vi "inputOLD.vi"(8 "error in":errorcluster, 9 "result allocation":T1, 10 "parameters":T1, 11 "module in":refnum<class "current tag file io module runtime.lvclass">) -> (0 "error out":errorcluster, 1 "results":T1, 2 "parameter allocation":T1, 3 "module out":refnum<class "current tag file io module runtime.lvclass">)   [LabVIEW 2013, in "current tag file io module runtime.lvclass"]
doc: "Provides an interface for information processing by a module at runtime. While this interface performs no operations, a child should provide an override which may process data in any manner necessary."
uses:
  current tag file io module runtime.lvclass
  <vilib>/NI/Tag Bus/table/data table.lvlib
  <vilib>/NI/Tag Bus/table/data polymorphs/read one/read Double.vi
  <vilib>/NI/Tag Bus/table/data polymorphs/write one/write Double.vi
  <vilib>/NI/Tag Bus/table/data polymorphs/read one/read Boolean.vi
  <vilib>/NI/Tag Bus/table/data polymorphs/write one/write Array of String.vi
  <vilib>/NI/Tag Bus/table/data polymorphs/read one/read Array of String.vi
  <vilib>/NI/Tag Bus/table/data polymorphs/read one/read Single.vi
  <vilib>/NI/Tag Bus/table/data polymorphs/write one/write Single.vi
  <vilib>/NI/Tag Bus/table/data polymorphs/read one/read I64.vi
  <vilib>/NI/Tag Bus/table/data polymorphs/write one/write I64.vi
  <vilib>/NI/Tag Bus/table/data polymorphs/read one/read I32.vi
  <vilib>/NI/Tag Bus/table/data polymorphs/write one/write I32.vi
  <vilib>/NI/Tag Bus/table/data polymorphs/read one/read I16.vi
  <vilib>/NI/Tag Bus/table/data polymorphs/write one/write I16.vi
  <vilib>/NI/Tag Bus/table/data polymorphs/read one/read I8.vi
  <vilib>/NI/Tag Bus/table/data polymorphs/write one/write I8.vi
  <vilib>/NI/Tag Bus/table/data polymorphs/read one/read U64.vi
  <vilib>/NI/Tag Bus/table/data polymorphs/write one/write U64.vi
  <vilib>/NI/Tag Bus/table/data polymorphs/read one/read U32.vi
  <vilib>/NI/Tag Bus/table/data polymorphs/write one/write U32.vi
  <vilib>/NI/Tag Bus/table/data polymorphs/read one/read U16.vi
  <vilib>/NI/Tag Bus/table/data polymorphs/write one/write U16.vi
  <vilib>/NI/Tag Bus/table/data polymorphs/read one/read U8.vi
  <vilib>/NI/Tag Bus/table/data polymorphs/write one/write U8.vi
  <vilib>/NI/Tag Bus/table/data polymorphs/write one/write Boolean.vi
  <vilib>/NI/Tag Bus/table/data polymorphs/read one/read String.vi
  <vilib>/NI/Tag Bus/table/data polymorphs/write one/write String.vi
  <vilib>/NI/Tag Bus/table/data polymorphs/read one/read Array of Double.vi
  <vilib>/NI/Tag Bus/table/data polymorphs/write one/write Array of Double.vi
  <vilib>/NI/Tag Bus/table/data polymorphs/read one/read Array of Single.vi
  <vilib>/NI/Tag Bus/table/data polymorphs/write one/write Array of Single.vi
  <vilib>/NI/Tag Bus/table/data polymorphs/read one/read Array of I64.vi
  <vilib>/NI/Tag Bus/table/data polymorphs/write one/write Array of I64.vi
  <vilib>/NI/Tag Bus/table/data polymorphs/read one/read Array of I32.vi
  <vilib>/NI/Tag Bus/table/data polymorphs/write one/write Array of I32.vi
  <vilib>/NI/Tag Bus/table/data polymorphs/read one/read Array of I16.vi
  <vilib>/NI/Tag Bus/table/data polymorphs/write one/write Array of I16.vi
  <vilib>/NI/Tag Bus/table/data polymorphs/read one/read Array of I8.vi
  <vilib>/NI/Tag Bus/table/data polymorphs/write one/write Array of I8.vi
  <vilib>/NI/Tag Bus/table/data polymorphs/read one/read Array of U64.vi
  <vilib>/NI/Tag Bus/table/data polymorphs/write one/write Array of U64.vi
  <vilib>/NI/Tag Bus/table/data polymorphs/read one/read Array of U32.vi
  <vilib>/NI/Tag Bus/table/data polymorphs/write one/write Array of U32.vi
  <vilib>/NI/Tag Bus/table/data polymorphs/read one/read Array of U16.vi
  <vilib>/NI/Tag Bus/table/data polymorphs/write one/write Array of U16.vi
  <vilib>/NI/Tag Bus/table/data polymorphs/read one/read Array of U8.vi
  <vilib>/NI/Tag Bus/table/data polymorphs/write one/write Array of U8.vi
  <vilib>/NI/Tag Bus/table/data polymorphs/read one/read Array of Boolean.vi
  <vilib>/NI/Tag Bus/table/data polymorphs/write one/write Array of Boolean.vi
  <vilib>/NI/Tag Bus/table/data table.ctl
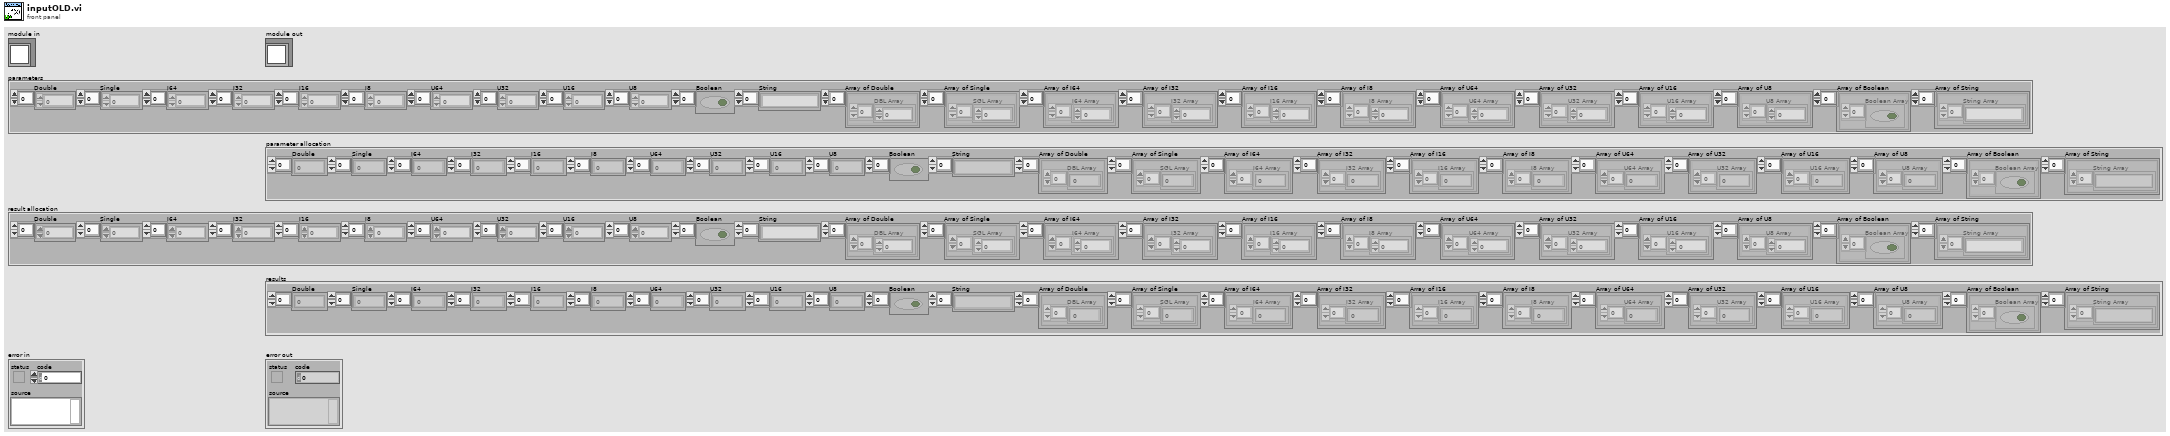
[diagram p1: front panel]
types:
  T1 = typedef "tag bus.lvlib/data table.lvlib/data table.ctl" = cluster{"Double":dbl[], "Single":sgl[], "I64":i64[], "I32":i32[], "I16":i16[], "I8":i8[], "U64":u64[], "U32":u32[], "U16":u16[], "U8":u8[], "Boolean":bool[], "String":string[], "Array of Double":cluster{"DBL Array":dbl[]}[], "Array of Single":cluster{"SGL Array":sgl[]}[], "Array of I64":cluster{"I64 Array":i64[]}[], "Array of I32":cluster{"I32 Array":i32[]}[], "Array of I16":cluster{"I16 Array":i16[]}[], "Array of I8":cluster{"I8 Array":i8[]}[], "Array of U64":cluster{"U64 Array":u64[]}[], "Array of U32":cluster{"U32 Array":u32[]}[], "Array of U16":cluster{"U16 Array":u16[]}[], "Array of U8":cluster{"U8 Array":u8[]}[], "Array of Boolean":cluster{"Boolean Array":bool[]}[], "Array of String":cluster{"String Array":string[]}[]}
  T2 = typedef "current tag file io module runtime.lvclass/current tag file io configuration.ctl" = cluster{"index":i32, "data type":T3, "refnum":refnum<file>}
  T3 = typedef "tag bus.lvlib/tag descriptor.lvclass/Data Type.ctl" = enum16{"Double", "Single", "I64", "I32", "I16", "I8", "U64", "U32", "U16", "U8", "Boolean", "String", "Array of Double", "Array of Single", "Array of I64", "Array of I32", "Array of I16", "Array of I8", "Array of U64", "Array of U32", "Array of U16", "Array of U8", "Array of Boolean", "Array of String"}
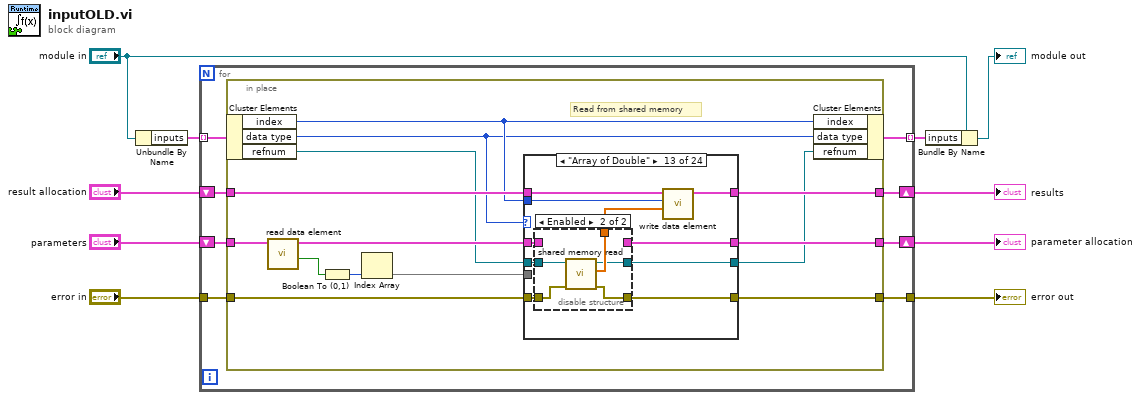
[diagram p0: block diagram]
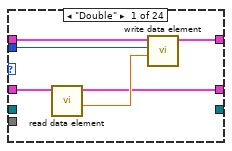
[diagram p2: hidden frame]
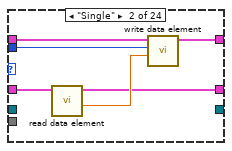
[diagram p3: hidden frame]
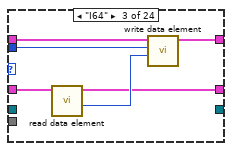
[diagram p4: hidden frame]
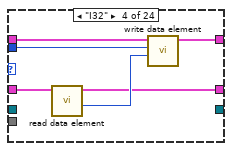
[diagram p5: hidden frame]
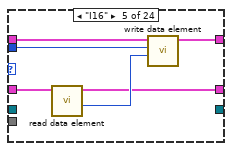
[diagram p6: hidden frame]
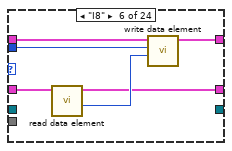
[diagram p7: hidden frame]
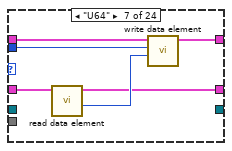
[diagram p8: hidden frame]
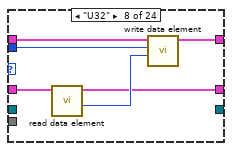
[diagram p9: hidden frame]
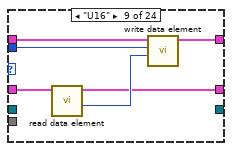
[diagram p10: hidden frame]
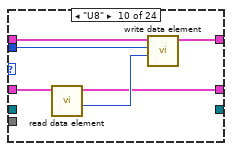
[diagram p11: hidden frame]
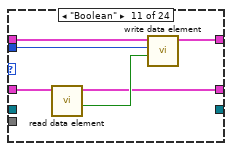
[diagram p12: hidden frame]
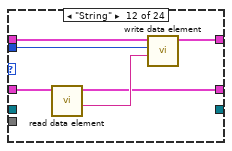
[diagram p13: hidden frame]
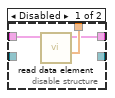
[diagram p14: hidden frame]
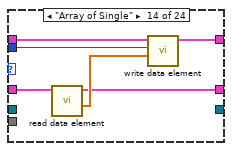
[diagram p15: hidden frame]
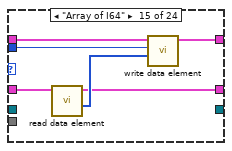
[diagram p16: hidden frame]
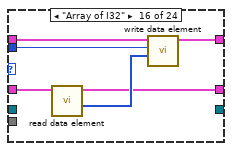
[diagram p17: hidden frame]
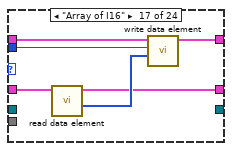
[diagram p18: hidden frame]
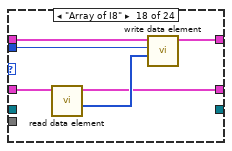
[diagram p19: hidden frame]
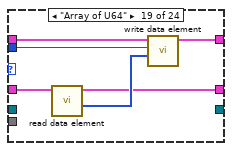
[diagram p20: hidden frame]
diagram:
  n1 = Unbundle By Name("module in") -> ("inputs"=w8:T2[])
  n2 = for {
    tunnel: w8 -> [w18] mode=indexing
    tunnel: [w17] -> w7 mode=indexing
    shift-right: [w13] -> w5
    shift-left: "parameters" -> [w16]
    shift-right: [w14] -> w3
    shift-left: "result allocation" -> [w15]
    tunnel: "error in" -> [w12]
    tunnel: [w11] -> w1
    n3 = in-place {
      in-place-border: w16 -> [w32]
      in-place-border: w15 -> [w31]
      in-place-border: [w30] -> w14
      in-place-border: [w25] -> w13
      in-place-border: w12 -> [w21]
      in-place-border: [w19] -> w11
      # "Read from shared memory"
      n4 = in-place-cluster #1(w18) -> ("index"=w24:i32, "data type"=w23:T3, "refnum"=w22:refnum<file>)
      n5 = call-poly <vilib>:"read data element.vi"("data table in"=w32) -> ("value"=w28:bool, "data table out"=w26:T1)  [unwired: 9 in]
      n6 = Boolean To (0,1)(Boolean=w28) -> (0, 1=w29:i16)
      n7 = Index Array(index=w29) -> (element=w27)  [unwired: 1 in]
      n8 = case shown="\"Array of Double\"" w23 {
        tunnel: w31 -> [w33 w39 w45 w51 w57 w63 w69 w75 w81 w87 w93 w99 w109 w123 w129 w135 w141 w147 w153 w159 w165 w171 w177 w183]
        tunnel: [w38 w44 w50 w56 w62 w68 w74 w80 w86 w92 w98 w104 w114 w128 w134 w140 w146 w152 w158 w164 w170 w176 w182 w188] -> w30
        tunnel: w27 -> [_ _ _ _ _ _ _ _ _ _ _ _ _ _ _ _ _ _ _ _ _ _ _ _]
        tunnel: w24 -> [w37 w43 w49 w55 w61 w67 w73 w79 w85 w91 w97 w103 w113 w127 w133 w139 w145 w151 w157 w163 w169 w175 w181 w187]
        tunnel: w26 -> [w35 w41 w47 w53 w59 w65 w71 w77 w83 w89 w95 w101 w111 w125 w131 w137 w143 w149 w155 w161 w167 w173 w179 w185]
        tunnel: [w34 w40 w46 w52 w58 w64 w70 w76 w82 w88 w94 w100 w110 w124 w130 w136 w142 w148 w154 w160 w166 w172 w178 w184] -> w25
        tunnel: w22 -> [_ _ _ _ _ _ _ _ _ _ _ _ w108 _ _ _ _ _ _ _ _ _ _ _]
        tunnel: w21 -> [_ _ _ _ _ _ _ _ _ _ _ _ w107 _ _ _ _ _ _ _ _ _ _ _]
        tunnel: [_ _ _ _ _ _ _ _ _ _ _ _ w106 _ _ _ _ _ _ _ _ _ _ _] -> w20
        tunnel: [_ _ _ _ _ _ _ _ _ _ _ _ w105 _ _ _ _ _ _ _ _ _ _ _] -> w19
        frame "Double" {
          n9 = call-poly <vilib>:"read data element.vi"("data table in"=w35) -> ("value"=w36:dbl, "data table out"=w34:T1)  [unwired: 9 in]
          n10 = call-poly <vilib>:"write data element.vi"("value"=w36, "index"=w37, "data table in"=w33) -> ("data table out"=w38:T1)  [unwired: 8 in]
        }
        frame "Single" {
          n11 = call-poly <vilib>:"read data element.vi"("data table in"=w41) -> ("value"=w42:sgl, "data table out"=w40:T1)  [unwired: 9 in]
          n12 = call-poly <vilib>:"write data element.vi"("value"=w42, "index"=w43, "data table in"=w39) -> ("data table out"=w44:T1)  [unwired: 8 in]
        }
        frame "I64" {
          n13 = call-poly <vilib>:"read data element.vi"("data table in"=w47) -> ("value"=w48:i64, "data table out"=w46:T1)  [unwired: 9 in]
          n14 = call-poly <vilib>:"write data element.vi"("value"=w48, "index"=w49, "data table in"=w45) -> ("data table out"=w50:T1)  [unwired: 8 in]
        }
        frame "I32" {
          n15 = call-poly <vilib>:"read data element.vi"("data table in"=w53) -> ("value"=w54:i32, "data table out"=w52:T1)  [unwired: 9 in]
          n16 = call-poly <vilib>:"write data element.vi"("value"=w54, "index"=w55, "data table in"=w51) -> ("data table out"=w56:T1)  [unwired: 8 in]
        }
        frame "I16" {
          n17 = call-poly <vilib>:"read data element.vi"("data table in"=w59) -> ("value"=w60:i16, "data table out"=w58:T1)  [unwired: 9 in]
          n18 = call-poly <vilib>:"write data element.vi"("value"=w60, "index"=w61, "data table in"=w57) -> ("data table out"=w62:T1)  [unwired: 8 in]
        }
        frame "I8" {
          n19 = call-poly <vilib>:"read data element.vi"("data table in"=w65) -> ("value"=w66:i8, "data table out"=w64:T1)  [unwired: 9 in]
          n20 = call-poly <vilib>:"write data element.vi"("value"=w66, "index"=w67, "data table in"=w63) -> ("data table out"=w68:T1)  [unwired: 8 in]
        }
        frame "U64" {
          n21 = call-poly <vilib>:"read data element.vi"("data table in"=w71) -> ("value"=w72:u64, "data table out"=w70:T1)  [unwired: 9 in]
          n22 = call-poly <vilib>:"write data element.vi"("value"=w72, "index"=w73, "data table in"=w69) -> ("data table out"=w74:T1)  [unwired: 8 in]
        }
        frame "U32" {
          n23 = call-poly <vilib>:"read data element.vi"("data table in"=w77) -> ("value"=w78:u32, "data table out"=w76:T1)  [unwired: 9 in]
          n24 = call-poly <vilib>:"write data element.vi"("value"=w78, "index"=w79, "data table in"=w75) -> ("data table out"=w80:T1)  [unwired: 8 in]
        }
        frame "U16" {
          n25 = call-poly <vilib>:"read data element.vi"("data table in"=w83) -> ("value"=w84:u16, "data table out"=w82:T1)  [unwired: 9 in]
          n26 = call-poly <vilib>:"write data element.vi"("value"=w84, "index"=w85, "data table in"=w81) -> ("data table out"=w86:T1)  [unwired: 8 in]
        }
        frame "U8" {
          n27 = call-poly <vilib>:"read data element.vi"("data table in"=w89) -> ("value"=w90:u8, "data table out"=w88:T1)  [unwired: 9 in]
          n28 = call-poly <vilib>:"write data element.vi"("value"=w90, "index"=w91, "data table in"=w87) -> ("data table out"=w92:T1)  [unwired: 8 in]
        }
        frame "Boolean" {
          n29 = call-poly <vilib>:"read data element.vi"("data table in"=w95) -> ("value"=w96:bool, "data table out"=w94:T1)  [unwired: 9 in]
          n30 = call-poly <vilib>:"write data element.vi"("value"=w96, "index"=w97, "data table in"=w93) -> ("data table out"=w98:T1)  [unwired: 8 in]
        }
        frame "String" {
          n31 = call-poly <vilib>:"read data element.vi"("data table in"=w101) -> ("value"=w102:string, "data table out"=w100:T1)  [unwired: 9 in]
          n32 = call-poly <vilib>:"write data element.vi"("value"=w102, "index"=w103, "data table in"=w99) -> ("data table out"=w104:T1)  [unwired: 8 in]
        }
        frame "Array of Double" {
          n33 = disable-structure shown="Enabled" {
            disable-tunnel: [w117 w122] -> w112
            disable-tunnel: w111 -> [w116 _]
            disable-tunnel: [w115 _] -> w110
            disable-tunnel: w108 -> [_ w121]
            disable-tunnel: w107 -> [_ w120]
            disable-tunnel: [_ w119] -> w106
            disable-tunnel: [_ w118] -> w105
            frame Disabled {
              n34 = call-poly <vilib>:"read data element.vi"("data table in"=w116) -> ("value"=w117:dbl[], "data table out"=w115:T1)  [unwired: 9 in]
            }
            frame Enabled {
              n35 = call "shared memory read.vi"("error in"=w120, "refnum in"=w121) -> ("error out"=w118:errorcluster, "Data Array out"=w122:dbl[], "refnum out"=w119:refnum<file>)  [unwired: 6 in, 1 out]
            }
          }
          n36 = call-poly <vilib>:"write data element.vi"("value"=w112, "index"=w113, "data table in"=w109) -> ("data table out"=w114:T1)  [unwired: 8 in]
        }
        frame "Array of Single" {
          n37 = call-poly <vilib>:"read data element.vi"("data table in"=w125) -> ("value"=w126:sgl[], "data table out"=w124:T1)  [unwired: 9 in]
          n38 = call-poly <vilib>:"write data element.vi"("value"=w126, "index"=w127, "data table in"=w123) -> ("data table out"=w128:T1)  [unwired: 8 in]
        }
        frame "Array of I64" {
          n39 = call-poly <vilib>:"read data element.vi"("data table in"=w131) -> ("value"=w132:i64[], "data table out"=w130:T1)  [unwired: 9 in]
          n40 = call-poly <vilib>:"write data element.vi"("value"=w132, "index"=w133, "data table in"=w129) -> ("data table out"=w134:T1)  [unwired: 8 in]
        }
        frame "Array of I32" {
          n41 = call-poly <vilib>:"read data element.vi"("data table in"=w137) -> ("value"=w138:i32[], "data table out"=w136:T1)  [unwired: 9 in]
          n42 = call-poly <vilib>:"write data element.vi"("value"=w138, "index"=w139, "data table in"=w135) -> ("data table out"=w140:T1)  [unwired: 8 in]
        }
        frame "Array of I16" {
          n43 = call-poly <vilib>:"read data element.vi"("data table in"=w143) -> ("value"=w144:i16[], "data table out"=w142:T1)  [unwired: 9 in]
          n44 = call-poly <vilib>:"write data element.vi"("value"=w144, "index"=w145, "data table in"=w141) -> ("data table out"=w146:T1)  [unwired: 8 in]
        }
        frame "Array of I8" {
          n45 = call-poly <vilib>:"read data element.vi"("data table in"=w149) -> ("value"=w150:i8[], "data table out"=w148:T1)  [unwired: 9 in]
          n46 = call-poly <vilib>:"write data element.vi"("value"=w150, "index"=w151, "data table in"=w147) -> ("data table out"=w152:T1)  [unwired: 8 in]
        }
        frame "Array of U64" {
          n47 = call-poly <vilib>:"read data element.vi"("data table in"=w155) -> ("value"=w156:u64[], "data table out"=w154:T1)  [unwired: 9 in]
          n48 = call-poly <vilib>:"write data element.vi"("value"=w156, "index"=w157, "data table in"=w153) -> ("data table out"=w158:T1)  [unwired: 8 in]
        }
        frame "Array of U32" {
          n49 = call-poly <vilib>:"read data element.vi"("data table in"=w161) -> ("value"=w162:u32[], "data table out"=w160:T1)  [unwired: 9 in]
          n50 = call-poly <vilib>:"write data element.vi"("value"=w162, "index"=w163, "data table in"=w159) -> ("data table out"=w164:T1)  [unwired: 8 in]
        }
        frame "Array of U16" {
          n51 = call-poly <vilib>:"read data element.vi"("data table in"=w167) -> ("value"=w168:u16[], "data table out"=w166:T1)  [unwired: 9 in]
          n52 = call-poly <vilib>:"write data element.vi"("value"=w168, "index"=w169, "data table in"=w165) -> ("data table out"=w170:T1)  [unwired: 8 in]
        }
        frame "Array of U8" {
          n53 = call-poly <vilib>:"read data element.vi"("data table in"=w173) -> ("value"=w174:u8[], "data table out"=w172:T1)  [unwired: 9 in]
          n54 = call-poly <vilib>:"write data element.vi"("value"=w174, "index"=w175, "data table in"=w171) -> ("data table out"=w176:T1)  [unwired: 8 in]
        }
        frame "Array of Boolean" {
          n55 = call-poly <vilib>:"read data element.vi"("data table in"=w179) -> ("value"=w180:bool[], "data table out"=w178:T1)  [unwired: 9 in]
          n56 = call-poly <vilib>:"write data element.vi"("value"=w180, "index"=w181, "data table in"=w177) -> ("data table out"=w182:T1)  [unwired: 8 in]
        }
        frame "Array of String" {
          n57 = call-poly <vilib>:"read data element.vi"("data table in"=w185) -> ("value"=w186:string[], "data table out"=w184:T1)  [unwired: 9 in]
          n58 = call-poly <vilib>:"write data element.vi"("value"=w186, "index"=w187, "data table in"=w183) -> ("data table out"=w188:T1)  [unwired: 8 in]
        }
      }
      n59 = in-place-cluster #1("index"=w24, "data type"=w23, "refnum"=w20) -> (w17:T2)
    }
  }
  "error out" <- w1
  "results" <- w3
  "parameter allocation" <- w5
  n60 = Bundle By Name(cluster="module in", "inputs"=w7) -> (→"module out":refnum<class "current tag file io module runtime.lvclass">)
